vi "Main.vi"() -> ()   [LabVIEW 2019]
panel:
  in  "stop":bool
  out "Salida":dbl
  in  "Entrada":dbl
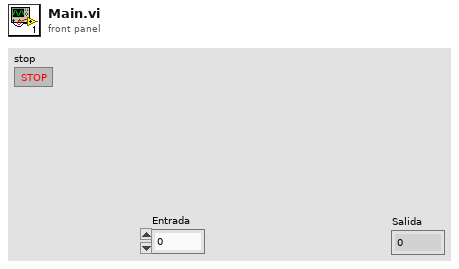
[diagram p1: front panel]
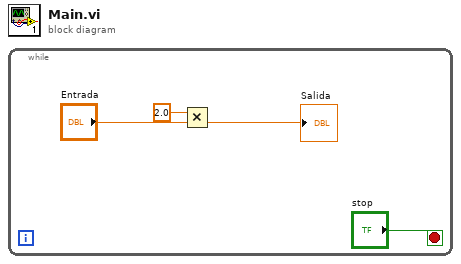
[diagram p0: block diagram]
diagram:
  n1 = while {
    stop <- "stop" stop-if-true
    n2 = Multiply(x=2.0, y="Entrada") -> (x*y=→"Salida":dbl)
  }
